vi "All_stats_labels.vi"() -> (0 "No of stats columns":i32[](array[numeric]), 3 "Stats labels":string[](array[string]))   [LabVIEW 2010]
uses:
  Controls/Inst_type.ctl
  Globals/Meas_global.vi
  Globals/Trav_pos_global.vi
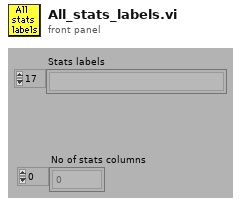
[diagram p1: front panel]
types:
  T1 = typedef "Tunnel_Coordinates.ctl" = enum16{"Work in Tunnel Coordinates", "Work in Model Coordinates"}
  T2 = typedef "Analysis_info_cluster.ctl" = cluster{"Colour":u32, "Inst type":T3, "Inst name":string, "Symbol":string, "Code name":string, "Extra Info":string, "Inst Array":T4, "Index":i32, "Voltage Index":i32, "Extra Titles":string[], "Extra Values":string[]}
  T3 = typedef "Inst_type.ctl" = enum16{"Propeller anemometer", "Raw voltage", "Pressure Transducer", "Pitot-static tube", "Preston tube", "Hot wire", "Cross wire 1", "Cross wire 2", "Generic Linear", "Generic Polynomial", "Generic BackPoly", "Fast FID", "Thermocouple", "Cold wire", "Pulsed Wire", "LDA Vel", "LDA Tran time", "LDA Arr time"}
  T4 = typedef "Instrument_Array.ctl" = enum16{"PWA", "LDA", "Analogue"}
  T5 = typedef "Analysis_type_cluster.ctl" = cluster{"Analysis type":T6, "Indicies":i32[], "Name":string, "Inst Array":T4, "Info index":i32}
  T6 = typedef "Analysis_type_Enum.ctl" = enum16{"Slow Response", "Fast Response", "Weighted Fast Response", "Fast FID", "Weighted Fast FID", "Cross Wire", "Weighted Cross Wire", "Weighted LDA"}
  T7 = enum16{"Mean only", "2nd Order Stats", "4th Order Stats"}
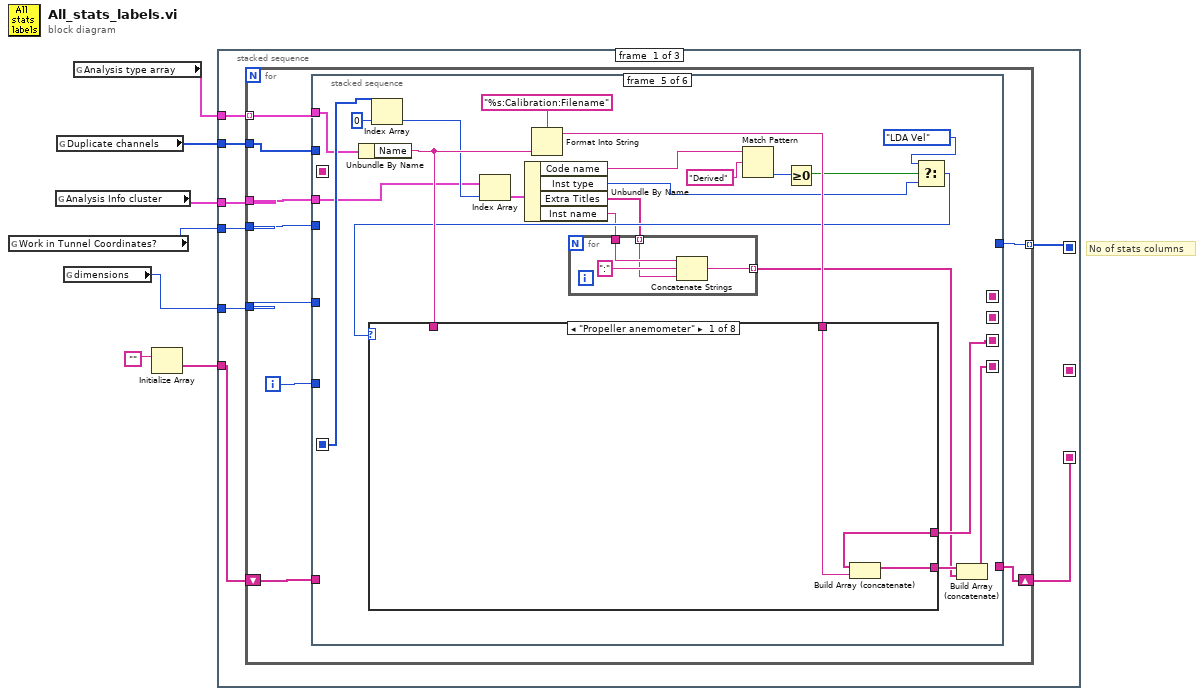
[diagram p0: block diagram]
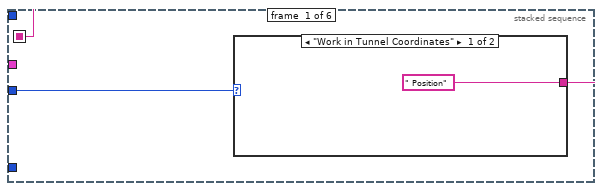
[diagram p2: hidden frame]
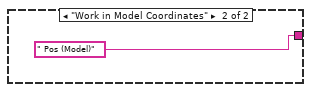
[diagram p3: hidden frame]
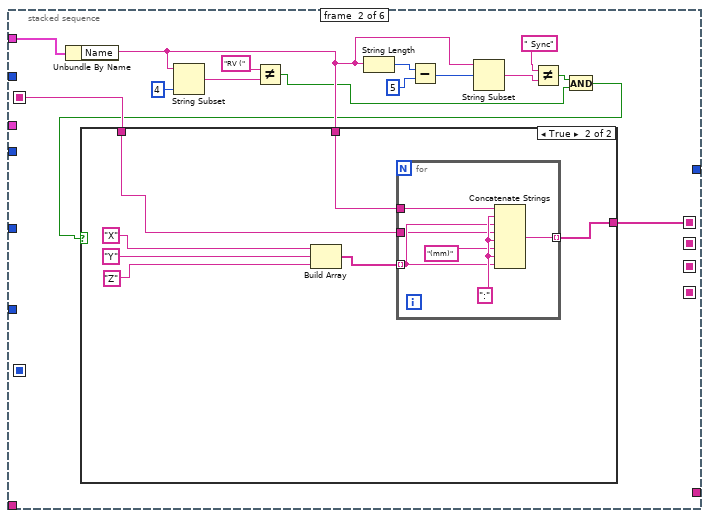
[diagram p4: hidden frame]
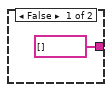
[diagram p5: hidden frame]
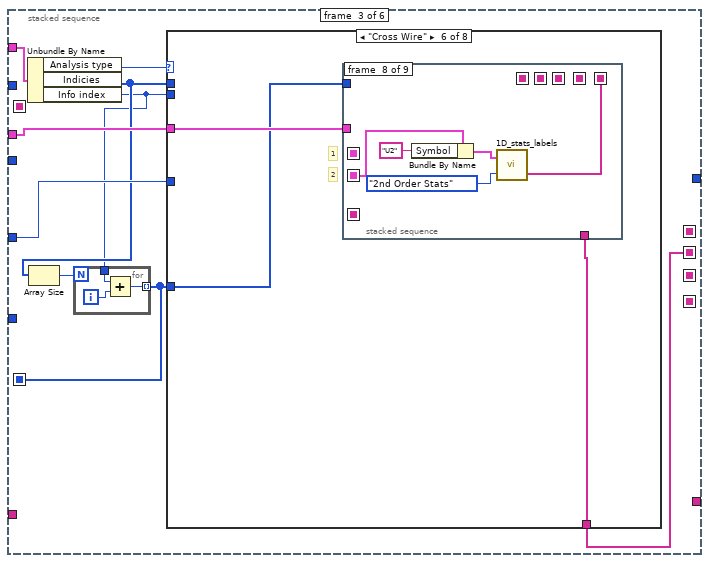
[diagram p6: hidden frame]
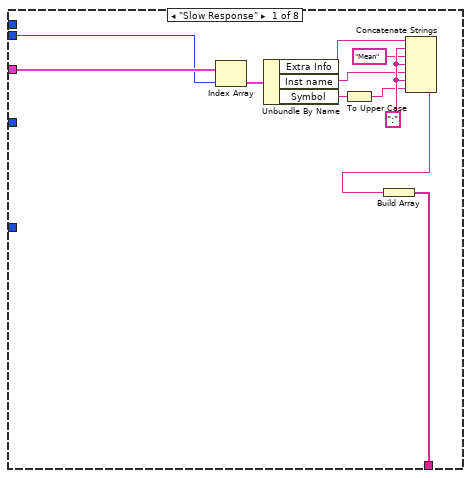
[diagram p7: hidden frame]
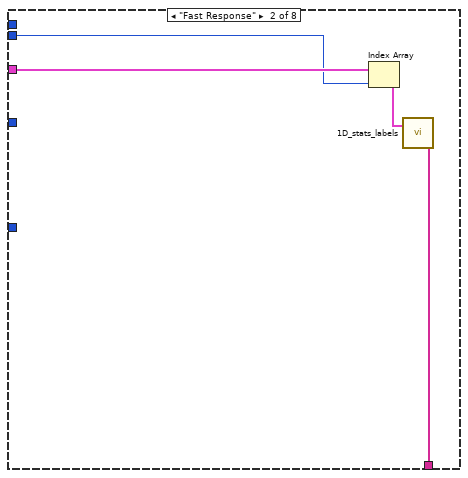
[diagram p8: hidden frame]
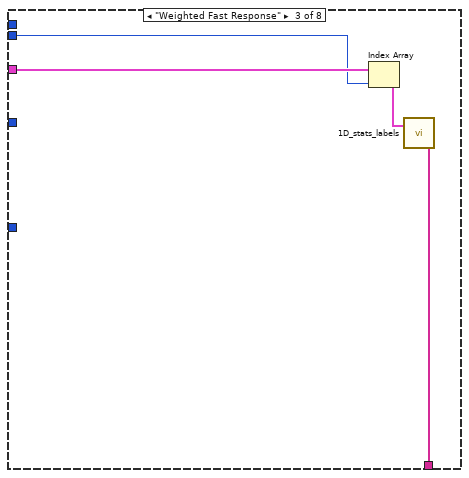
[diagram p9: hidden frame]
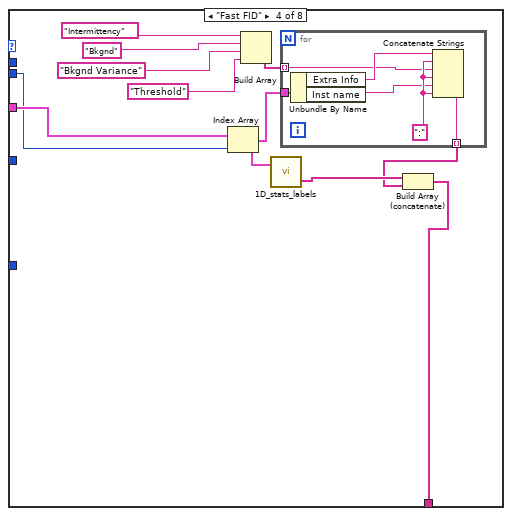
[diagram p10: hidden frame]
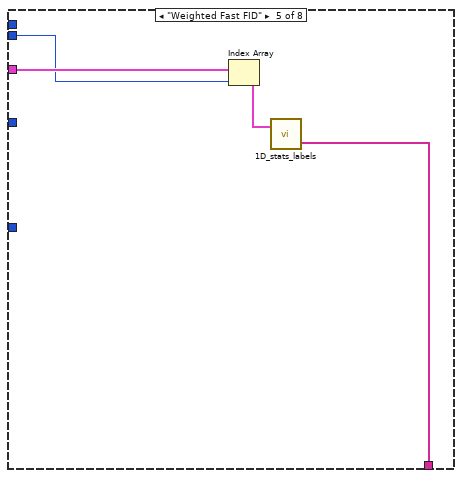
[diagram p11: hidden frame]
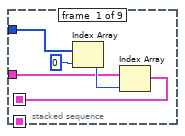
[diagram p12: hidden frame]
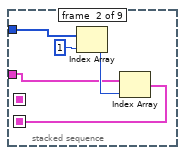
[diagram p13: hidden frame]
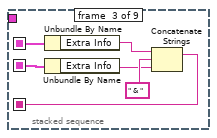
[diagram p14: hidden frame]
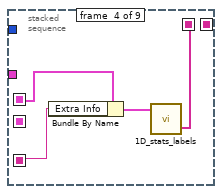
[diagram p15: hidden frame]
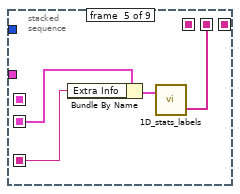
[diagram p16: hidden frame]
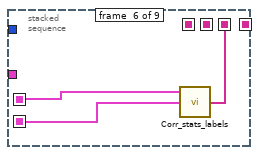
[diagram p17: hidden frame]
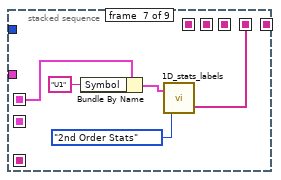
[diagram p18: hidden frame]
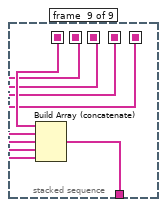
[diagram p19: hidden frame]
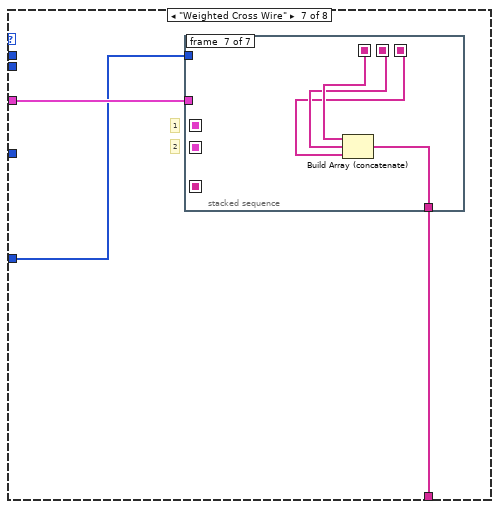
[diagram p20: hidden frame]
diagram:
  # "No of stats columns"
  n1 = global read "Trav_pos_global.vi" "Work in Tunnel Coordinates?"() -> (w2:T1)
  n2 = global read "Meas_global.vi" "Analysis Info cluster"() -> (w3:T2[])
  n3 = global read "Meas_global.vi" "Duplicate channels"() -> (w1:i32[])
  n4 = global read "Meas_global.vi" "dimensions"() -> (w4:enum16{"1D", "2D"})
  n5 = global read "Meas_global.vi" "Analysis type array"() -> (w7:T5[])
  n6 = Initialize Array("") -> (w5:string[])  [unwired: 1 out]
  n7 = stacked-sequence {
    seq-local: [w12 _ _] -> [_ _ w376]
    seq-local: [_ w358 _] -> [_ _ w373]
    seq-local: [w11 _ _] -> [_ _ w374]
    tunnel: w3 -> [w15 w359 _]
    tunnel: w7 -> [w14 _ _]
    tunnel: w5 -> [w10 _ _]
    tunnel: w4 -> [w13 _ _]
    tunnel: w2 -> [w9 _ _]
    tunnel: w1 -> [w8 _ _]
    frame #0 {
      n8 = for {
        shift-right: [w16] -> w12
        shift-left: w10 -> [w17]
        tunnel: w14 -> [w20] mode=indexing
        tunnel: w15 -> [w23]
        tunnel: w13 -> [w24]
        tunnel: [w22] -> w11 mode=indexing
        tunnel: w9 -> [w21]
        tunnel: w8 -> [w18]
        i -> [w19]
        n9 = stacked-sequence {
          seq-local: [_ _ w63 _ _ _] -> [_ _ _ w264 _ _]
          seq-local: [_ w41 _ _ _ _] -> [_ _ _ _ _ w345]
          seq-local: [w25 _ _ _ _ _] -> [_ w42 _ _ _ _]
          seq-local: [_ _ _ w263 _ _] -> [_ _ _ _ w303 _]
          seq-local: [_ _ _ _ w291 _] -> [_ _ _ _ _ w338]
          seq-local: [_ _ w58 _ _ _] -> [_ _ _ w262 w306 _]
          tunnel: w20 -> [_ w43 w66 _ w305 _]
          tunnel: w24 -> [_ _ w64 _ _ _]
          tunnel: w23 -> [_ _ w62 w265 w290 _]
          tunnel: [_ _ _ _ _ w344] -> w22
          tunnel: w21 -> [w26 _ _ _ _ _]
          tunnel: w19 -> [_ _ _ _ _ w343]
          tunnel: w18 -> [_ _ _ _ _ w342]
          tunnel: w17 -> [_ _ _ _ _ w341]
          tunnel: [_ _ _ _ _ w340] -> w16
          frame #0 {
            n10 = case shown="\"Work in Tunnel Coordinates\"" w26 {
              tunnel: [" Position" " Pos (Model)"] -> w25
              frame "Work in Tunnel Coordinates" {
              }
              frame "Work in Model Coordinates" {
              }
            }
          }
          frame #1 {
            n11 = Unbundle By Name(w43) -> ("Name"=w35:string)
            n12 = String Subset(string=w35, length (rest)=4 ("length (rest)")) -> (substring=w33:string)  [unwired: 1 out]
            n13 = Not Equal?(x="RV (", y=w33) -> (x != y?=w30:bool)
            n14 = String Length(string=w35) -> (length=w40:i32)
            n15 = Subtract(x=w40, y=5) -> (x-y=w38:i32)
            n16 = String Subset(string=w35, offset (0)=w38) -> (substring=w36:string)  [unwired: 1 out]
            n17 = Not Equal?(x=" Sync" ("substring"), y=w36) -> (x != y?=w31:bool)
            n18 = And(x=w31, y=w30) -> (x .and. y?=w29:bool)
            n19 = case shown="True" w29 {
              tunnel: w35 -> [_ w47]
              tunnel: w42 -> [_ w46]
              tunnel: [string[] [] w45] -> w41
              frame False {
              }
              frame True {
                n20 = Build Array("X", "Y", "Z") -> (w48:string[])
                n21 = for {
                  tunnel: w48 -> [w55] mode=indexing
                  tunnel: w47 -> [w57]
                  tunnel: [w53] -> w45 mode=indexing
                  tunnel: w46 -> [w52]
                  w56 = ":" ("Substring")
                  n22 = Concatenate Strings(w57, w56, w55, w52, w56, "(mm)", w56, w55) -> (w53:string)
                }
              }
            }
          }
          frame #2 {
            n23 = Unbundle By Name(w66) -> ("Analysis type"=w65:T6, "Indicies"=w60:i32[], "Info index"=w59:i32)
            n24 = Array Size(array=w60) -> (size(s)=w61:i32)
            n25 = for {
              N: w61 -> [_]
              tunnel: w59 -> [w68]
              tunnel: [w67] -> w58 mode=indexing
              i -> [w69]
              n26 = Add(x=w68, y=w69) -> (x+y=w67:i32)
            }
            n27 = case shown="\"Cross Wire\"" w65 {
              tunnel: w60 -> [_ _ _ _ _ _ _ _]
              tunnel: [w71 w83 w87 w96 w107 w112 w158 w193] -> w63
              tunnel: w64 -> [_ _ _ _ _ _ _ w192]
              tunnel: w62 -> [w80 w82 w86 w94 w109 w111 w157 w191]
              tunnel: w59 -> [w70 w81 w85 w89 w106 _ _ _]
              tunnel: w58 -> [_ _ _ _ _ w110 w156 w190]
              frame "Slow Response" {
                w79 = ":" ("Substring")
                n28 = Index Array(array=w80, index=w70) -> (element=w73:T2)
                n29 = Unbundle By Name(w73) -> ("Extra Info"=w78:string, "Inst name"=w76:string, "Symbol"=w75:string)
                n30 = To Upper Case(1:w75) -> (0:w74:string)
                n31 = Concatenate Strings(w78, w79, "Mean", w79, w76, w79, w74) -> (w72:string)
                n32 = Build Array(w72) -> (w71:string[])
              }
              frame "Fast Response" {
                n33 = Index Array(array=w82, index=w81) -> (element=w84:T2)
                n34 = call "1D_stats_labels.vi"("Analysis Info Cluster"=w84) -> ("Output"=w83:string[])  [unwired: 1 in, 1 out]
              }
              frame "Weighted Fast Response" {
                n35 = Index Array(array=w86, index=w85) -> (element=w88:T2)
                n36 = call "1D_stats_labels.vi"("Analysis Info Cluster"=w88) -> ("Output"=w87:string[])  [unwired: 1 in, 1 out]
              }
              frame "Fast FID" {
                n37 = Index Array(array=w94, index=w89) -> (element=w99:T2)
                n38 = Build Array("Intermittency", "Bkgnd", "Bkgnd Variance", "Threshold") -> (w95:string[])
                n39 = call "1D_stats_labels.vi"("Analysis Info Cluster"=w99) -> ("Output"=w98:string[])  [unwired: 1 in, 1 out]
                n40 = for {
                  tunnel: w99 -> [w102]
                  tunnel: [w101] -> w97 mode=indexing
                  tunnel: w95 -> [w100] mode=indexing
                  w105 = ":" ("Substring")
                  n41 = Unbundle By Name(w102) -> ("Extra Info"=w104:string, "Inst name"=w103:string)
                  n42 = Concatenate Strings(w104, w105, w100, w105, w103, w105) -> (w101:string)
                }
                n43 = Build Array (concatenate)(w98, w97) -> (w96:string[])
              }
              frame "Weighted Fast FID" {
                n44 = Index Array(array=w109, index=w106) -> (element=w108:T2)
                n45 = call "1D_stats_labels.vi"("Analysis Info Cluster"=w108) -> ("Output"=w107:string[])  [unwired: 1 in, 1 out]
              }
              frame "Cross Wire" {
                # "2"
                # "1"
                n46 = stacked-sequence {
                  seq-local: [_ _ _ w132 _ _ _ _ _] -> [_ _ _ _ _ _ _ _ w155]
                  seq-local: [_ _ _ _ w136 _ _ _ _] -> [_ _ _ _ _ _ _ _ w154]
                  seq-local: [_ _ _ _ _ w139 _ _ _] -> [_ _ _ _ _ _ _ _ w153]
                  seq-local: [_ _ _ _ _ _ w144 _ _] -> [_ _ _ _ _ _ _ _ w152]
                  seq-local: [_ _ _ _ _ _ _ w149 _] -> [_ _ _ _ _ _ _ _ w151]
                  seq-local: [w113 _ _ _ _ _ _ _ _] -> [_ _ w128 w131 _ w138 w142 _ _]
                  seq-local: [_ w118 _ _ _ _ _ _ _] -> [_ _ w127 _ w134 w137 _ w146 _]
                  seq-local: [_ _ w126 _ _ _ _ _ _] -> [_ _ _ w130 w133 _ _ _ _]
                  tunnel: [_ _ _ _ _ _ _ _ w150] -> w112
                  tunnel: w110 -> [w115 w120 _ _ _ _ _ _ _]
                  tunnel: w111 -> [w114 w119 _ _ _ _ _ _ _]
                  frame #0 {
                    n47 = Index Array(array=w115, index=0) -> (element=w117:i32)
                    n48 = Index Array(array=w114, index=w117) -> (element=w113:T2)
                  }
                  frame #1 {
                    n49 = Index Array(array=w120, index=1) -> (element=w122:i32)
                    n50 = Index Array(array=w119, index=w122) -> (element=w118:T2)
                  }
                  frame #2 {
                    n51 = Unbundle By Name(w128) -> ("Extra Info"=w123:string)
                    n52 = Unbundle By Name(w127) -> ("Extra Info"=w124:string)
                    n53 = Concatenate Strings(w123, " & ", w124) -> (w126:string)
                  }
                  frame #3 {
                    n54 = Bundle By Name(cluster=w131, "Extra Info"=w130) -> (w129:T2)
                    n55 = call "1D_stats_labels.vi"("Analysis Info Cluster"=w129) -> ("Output"=w132:string[])  [unwired: 1 in, 1 out]
                  }
                  frame #4 {
                    n56 = Bundle By Name(cluster=w134, "Extra Info"=w133) -> (w135:T2)
                    n57 = call "1D_stats_labels.vi"("Analysis Info Cluster"=w135) -> ("Output"=w136:string[])  [unwired: 1 in, 1 out]
                  }
                  frame #5 {
                    n58 = call "Corr_stats_labels.vi"("Inst 2 Units"=w137, "Inst 1 Units"=w138) -> ("Output"=w139:string[])  [unwired: 1 in]
                  }
                  frame #6 {
                    n59 = Bundle By Name(cluster=w142, "Symbol"="U1") -> (w141:T2)
                    n60 = call "1D_stats_labels.vi"("Mode selector"=T7."2nd Order Stats", "Analysis Info Cluster"=w141) -> ("Output"=w144:string[])  [unwired: 1 out]
                  }
                  frame #7 {
                    n61 = Bundle By Name(cluster=w146, "Symbol"="U2") -> (w145:T2)
                    n62 = call "1D_stats_labels.vi"("Mode selector"=T7."2nd Order Stats", "Analysis Info Cluster"=w145) -> ("Output"=w149:string[])  [unwired: 1 out]
                  }
                  frame #8 {
                    n63 = Build Array (concatenate)(w155, w154, w153, w152, w151) -> (w150:string[])
                  }
                }
              }
              frame "Weighted Cross Wire" {
                # "2"
                # "1"
                n64 = stacked-sequence {
                  seq-local: [_ _ _ w178 _ _ _] -> [_ _ _ _ _ _ w189]
                  seq-local: [_ _ _ _ w182 _ _] -> [_ _ _ _ _ _ w188]
                  seq-local: [_ _ _ _ _ w185 _] -> [_ _ _ _ _ _ w187]
                  seq-local: [w159 _ _ _ _ _ _] -> [_ _ w174 w177 _ w184 _]
                  seq-local: [_ w164 _ _ _ _ _] -> [_ _ w173 _ w180 w183 _]
                  seq-local: [_ _ w172 _ _ _ _] -> [_ _ _ w176 w179 _ _]
                  tunnel: [_ _ _ _ _ _ w186] -> w158
                  tunnel: w156 -> [w161 w166 _ _ _ _ _]
                  tunnel: w157 -> [w160 w165 _ _ _ _ _]
                  frame #0 {
                    n65 = Index Array(array=w161, index=0) -> (element=w163:i32)
                    n66 = Index Array(array=w160, index=w163) -> (element=w159:T2)
                  }
                  frame #1 {
                    n67 = Index Array(array=w166, index=1) -> (element=w168:i32)
                    n68 = Index Array(array=w165, index=w168) -> (element=w164:T2)
                  }
                  frame #2 {
                    n69 = Unbundle By Name(w174) -> ("Extra Info"=w169:string)
                    n70 = Unbundle By Name(w173) -> ("Extra Info"=w170:string)
                    n71 = Concatenate Strings(w169, " & ", w170) -> (w172:string)
                  }
                  frame #3 {
                    n72 = Bundle By Name(cluster=w177, "Extra Info"=w176) -> (w175:T2)
                    n73 = call "1D_stats_labels.vi"("Analysis Info Cluster"=w175) -> ("Output"=w178:string[])  [unwired: 1 in, 1 out]
                  }
                  frame #4 {
                    n74 = Bundle By Name(cluster=w180, "Extra Info"=w179) -> (w181:T2)
                    n75 = call "1D_stats_labels.vi"("Analysis Info Cluster"=w181) -> ("Output"=w182:string[])  [unwired: 1 in, 1 out]
                  }
                  frame #5 {
                    n76 = call "Corr_stats_labels.vi"("Inst 2 Units"=w183, "Inst 1 Units"=w184) -> ("Output"=w185:string[])  [unwired: 1 in]
                  }
                  frame #6 {
                    n77 = Build Array (concatenate)(w189, w188, w187) -> (w186:string[])
                  }
                }
              }
              frame "Weighted LDA" {
                n78 = case shown="\"2D\"" w192 {
                  tunnel: [w196 w221] -> w193
                  tunnel: w190 -> [w195 w220]
                  tunnel: w191 -> [w194 w219]
                  frame "1D" {
                    n79 = stacked-sequence {
                      seq-local: [w198 _ _] -> [_ _ w218]
                      seq-local: [_ w204 _] -> [_ _ w217]
                      tunnel: [_ _ w216] -> w196
                      tunnel: w195 -> [w199 w208 _]
                      tunnel: w194 -> [w197 w203 _]
                      frame #0 {
                        n80 = Index Array(array=w199, index=0) -> (element=w201:i32)
                        n81 = Index Array(array=w197, index=w201) -> (element=w202:T2)
                        n82 = call "1D_stats_labels.vi"("Analysis Info Cluster"=w202) -> ("Output"=w198:string[])  [unwired: 1 in, 1 out]
                      }
                      frame #1 {
                        n83 = Split 1D Array(array=w208, index=2) -> (second subarray=w206:i32[])  [unwired: 1 out]
                        n84 = for {
                          tunnel: w206 -> [w214] mode=indexing
                          shift-right: [w211] -> w204
                          shift-left: string[] [] -> [w213]
                          tunnel: w203 -> [w210]
                          n85 = Index Array(array=w210, index=w214) -> (element=w215:T2)
                          n86 = call "1D_stats_labels.vi"("Mode selector"=T7."Mean only", "Analysis Info Cluster"=w215) -> ("Output"=w212:string[])  [unwired: 1 out]
                          n87 = Build Array (concatenate)(w213, w212) -> (w211:string[])
                        }
                      }
                      frame #2 {
                        n88 = Build Array (concatenate)(w218, w217) -> (w216:string[])
                      }
                    }
                  }
                  frame "2D" {
                    n89 = stacked-sequence {
                      seq-local: [w223 _ _ _ _] -> [_ _ _ _ w260]
                      seq-local: [_ w229 _ _ _] -> [_ _ _ _ w259]
                      seq-local: [_ _ w235 _ _] -> [_ _ _ _ w258]
                      seq-local: [_ _ _ w244 _] -> [_ _ _ _ w257]
                      tunnel: [_ _ _ _ w256] -> w221
                      tunnel: w220 -> [w224 w230 w238 w248 _]
                      tunnel: w219 -> [w222 w228 w234 w243 _]
                      frame #0 {
                        n90 = Index Array(array=w224, index=0) -> (element=w226:i32)
                        n91 = Index Array(array=w222, index=w226) -> (element=w227:T2)
                        n92 = call "1D_stats_labels.vi"("Analysis Info Cluster"=w227) -> ("Output"=w223:string[])  [unwired: 1 in, 1 out]
                      }
                      frame #1 {
                        n93 = Index Array(array=w230, index=1) -> (element=w232:i32)
                        n94 = Index Array(array=w228, index=w232) -> (element=w233:T2)
                        n95 = call "1D_stats_labels.vi"("Analysis Info Cluster"=w233) -> ("Output"=w229:string[])  [unwired: 1 in, 1 out]
                      }
                      frame #2 {
                        n96 = Index Array(array=w238, index=0) -> (element=w241:i32)
                        n97 = Index Array(array=w238, index=1) -> (element=w237:i32)
                        n98 = Index Array(array=w234, index=w241) -> (element=w242:T2)
                        n99 = Index Array(array=w234, index=w237) -> (element=w236:T2)
                        n100 = call "Corr_stats_labels.vi"("Inst 2 Units"=w236, "Inst 1 Units"=w242) -> ("Output"=w235:string[])  [unwired: 1 in]
                      }
                      frame #3 {
                        n101 = Split 1D Array(array=w248, index=2) -> (second subarray=w246:i32[])  [unwired: 1 out]
                        n102 = for {
                          tunnel: w246 -> [w254] mode=indexing
                          shift-right: [w251] -> w244
                          shift-left: string[] [] -> [w253]
                          tunnel: w243 -> [w250]
                          n103 = Index Array(array=w250, index=w254) -> (element=w255:T2)
                          n104 = call "1D_stats_labels.vi"("Mode selector"=T7."Mean only", "Analysis Info Cluster"=w255) -> ("Output"=w252:string[])  [unwired: 1 out]
                          n105 = Build Array (concatenate)(w253, w252) -> (w251:string[])
                        }
                      }
                      frame #4 {
                        n106 = Build Array (concatenate)(w260, w259, w258, w257) -> (w256:string[])
                      }
                    }
                  }
                }
              }
            }
          }
          frame #3 {
            n107 = global read "Meas_global.vi" "Timescales (s)"() -> (w261:dbl[])
            n108 = for {
              tunnel: w261 -> [w269]
              tunnel: w262 -> [w266] mode=indexing
              shift-right: [w270] -> w263
              shift-left: w264 -> [w272]
              tunnel: w265 -> [w271]
              n109 = Index Array(array=w269, index=w266) -> (element=w268:dbl)
              n110 = Not A Number/Path/Refnum?(number/path/refnum=w268) -> (NaN/Path/Refnum?=w267:bool)
              n111 = case shown="False" w267 {
                tunnel: w272 -> [w285 w286]
                tunnel: [w284 w286] -> w270
                tunnel: w266 -> [w282 _]
                tunnel: w271 -> [w283 _]
                frame False {
                  n112 = Index Array(array=w283, index=w282) -> (element=w281:T2)
                  n113 = Unbundle By Name(w281) -> ("Inst name"=w277:string)
                  n114 = Format Into String(format string="%s:Standard Error:in Mean:Not %%", w277) -> (resulting string=w279:string)  [unwired: 2 in, 1 out]
                  n115 = Format Into String(format string="%s:Standard Error:in Variance:Not %%", w277) -> (resulting string=w275:string)  [unwired: 2 in, 1 out]
                  n116 = Format Into String(format string="%s:Timescale Estimate:Integrated to 25%%:(s)", w277) -> (resulting string=w273:string)  [unwired: 2 in, 1 out]
                  n117 = Build Array(w279, w275, w273) -> (w278:string[])
                  n118 = Build Array (concatenate)(w285, w278) -> (w284:string[])
                }
                frame True {
                }
              }
            }
          }
          frame #4 {
            n119 = Unbundle By Name(w305) -> ("Name"=w301:string)
            n120 = Index Array(array=w306, index=0 ("Index")) -> (element=w300:i32)
            n121 = Index Array(array=w290, index=w300) -> (element=w308:T2)
            n122 = Unbundle By Name(w308) -> ("Code name"=w294:string, "Inst type"=w298:T3, "Extra Titles"=w288:string[], "Inst name"=w289:string)
            n123 = Format Into String(format string="%s:Calibration:Filename" ("Format String"), w301) -> (resulting string=w302:string)  [unwired: 2 in, 1 out]
            n124 = for {
              tunnel: w289 -> [w312]
              tunnel: w288 -> [w310] mode=indexing
              tunnel: [w309] -> w287 mode=indexing
              n125 = Concatenate Strings(w312, ":" ("string"), w310) -> (w309:string)
            }
            n126 = Match Pattern(string=w294, regular expression="Derived") -> (offset past match=w295:i32)  [unwired: 4 out]
            n127 = Greater Or Equal To 0?(x=w295) -> (x >= 0?=w293:bool)
            n128 = Select(t=Inst_type."LDA Vel" ("Inst type"), s=w293, f=w298) -> (s? t:f=w297:T3)
            n129 = case shown="\"Propeller anemometer\"" w297 {
              tunnel: [w315 w318 w321 w327 w330 w334 w336 w337] -> w292
              tunnel: w303 -> [w314 w317 w320 w329 w332 w335 w336 w337]
              tunnel: w302 -> [w313 w316 w319 w328 w331 w333 _ _]
              tunnel: w301 -> [_ _ _ w324 _ _ _ _]
              frame "Propeller anemometer" {
                n130 = Build Array (concatenate)(w314, w313) -> (w315:string[])
              }
              frame "Preston tube" {
                n131 = Build Array (concatenate)(w317, w316) -> (w318:string[])
              }
              frame "Pressure Transducer" {
                n132 = Build Array (concatenate)(w320, w319) -> (w321:string[])
              }
              frame "Generic Linear", Default {
                n133 = Format Into String(format string="%s:Calibration:Interval:Minutes" ("Format String"), w324) -> (resulting string=w322:string)  [unwired: 2 in, 1 out]
                n134 = Format Into String(format string="%s:Calibration:Drift:%%" ("Format String"), w324) -> (resulting string=w323:string)  [unwired: 2 in, 1 out]
                n135 = Build Array (concatenate)(w329, w328, w323, w322) -> (w327:string[])
              }
              frame "Pulsed Wire" {
                n136 = Build Array (concatenate)(w332, w331) -> (w330:string[])
              }
              frame "Pitot-static tube" {
                n137 = Build Array (concatenate)(w335, w333) -> (w334:string[])
              }
              frame "Raw voltage" {
              }
              frame "LDA Vel" {
              }
            }
            n138 = Build Array (concatenate)(w292, w287) -> (w291:string[])
          }
          frame #5 {
            n139 = Search 1D Array(1D array=w342, element=w343) -> (index of element=w339:i32)  [unwired: 1 out]
            n140 = case shown="0" w339 {
              tunnel: w345 -> [w350 w356 _]
              tunnel: w338 -> [w349 w355 _]
              tunnel: w341 -> [w348 w354 w357]
              tunnel: [w347 w351 w357] -> w340
              frame -1 {
                n141 = Build Array (concatenate)(w350, w349) -> (w346:string[])
                n142 = Build Array (concatenate)(w348, w346) -> (w347:string[])
              }
              frame 0 {
                n143 = Build Array (concatenate)("Duplicated:Instrument:Name:", w356, w355) -> (w353:string[])
                n144 = Build Array (concatenate)(w354, w353) -> (w351:string[])
              }
              frame 1, Default {
              }
            }
            n145 = Array Size(array=w338) -> (size(s)=w344:i32)
          }
        }
      }
    }
    frame #1 {
      n146 = global read "Meas_global.vi" "correlate"() -> (w360:i32[][])
      n147 = for {
        shift-right: [w371] -> w358
        shift-left: string[] [] -> [w372]
        tunnel: w360 -> [w365] mode=indexing
        tunnel: w359 -> [w364]
        n148 = Index Array(array=w365, index=0) -> (element=w369:i32)
        n149 = Index Array(array=w365, index=1) -> (element=w367:i32)
        n150 = Index Array(array=w364, index=w369) -> (element=w363:T2)
        n151 = Index Array(array=w364, index=w367) -> (element=w362:T2)
        n152 = call "Corr_stats_labels.vi"("Inst 2 Units"=w362, "Inst 1 Units"=w363) -> ("Output"=w370:string[])  [unwired: 1 in]
        n153 = Build Array (concatenate)(w372, w370) -> (w371:string[])
      }
    }
    frame #2 {
      n154 = Build Array (concatenate)(w376, w373) -> (→"Stats labels":string[])
      "No of stats columns" <- w374
    }
  }
